vi "ExGlobalSetVar.vi"() -> ()   [LabVIEW 2010]
uses:
  Open-Close/CamHandle.vi
panel:
  in  "Value To Set":dbl format="%.2f"
  in  "Parameter ID":i32 min=0 step=1
  out "error out":errorcluster
  in  "error in (no error)":errorcluster
  # "ExGlobalSetVar:\nThis example allows the setting of a camera variable using a previously opened global camera handle."
  # "NOTICE\n\nTHIS VI USES A GLOBAL CAMERA HANDLE\n\nTHE VI EXOPENGLOBALCAM.VI MUST BE\nRUN AT THE START OF THE WORK SESSION.\nTHE CAMERA WILL REMAIN OPENED.\n\nTHE VI EXCLOSEGLOBALCAM.VI MUST\nBE RUN BEFORE LEAVING LABVIEW."
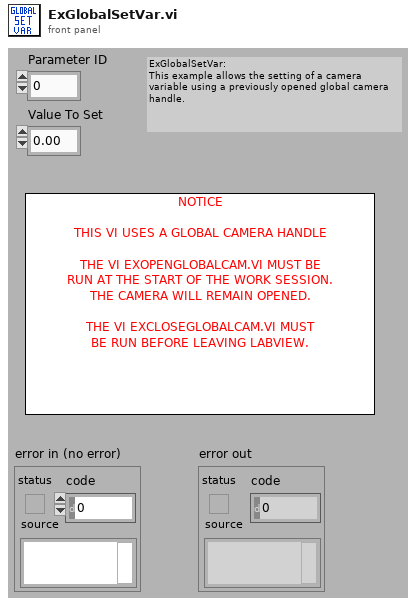
[diagram p1: front panel]
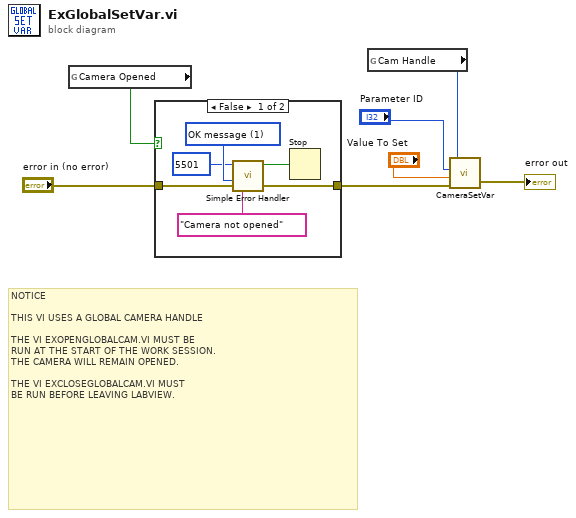
[diagram p0: block diagram]
diagram:
  # "NOTICE\n\nTHIS VI USES A GLOBAL CAMERA HANDLE\n\nTHE VI EXOPENGLOBALCAM.VI MUST BE\nRUN AT THE START OF THE WORK SESSION.\nTHE CAMERA WILL REMAIN OPENED.\n\nTHE VI EXCLOSEGLOBALCAM.VI MUST\nBE RUN BEFORE LEAVING LABVIEW."
  n1 = global read "CamHandle.vi" "Camera Opened"() -> (w4:bool)
  n2 = case shown="False" w4 {
    tunnel: "error in (no error)" -> [w12 w14]
    tunnel: [w11 w14] -> w5
    frame False {
      w13 = u16 1 items=["no dialog", "OK message", "continue or stop message"] ("type of dialog (OK msg:1)")
      n3 = call <vilib>:"Simple Error Handler.vi"("error code (no error:0)"=5501, "error source (\" \")"="Camera not opened", "type of dialog (OK msg:1)"=w13, "error in (no error)"=w12) -> ("error?"=w9:bool, "error out"=w11:errorcluster)  [unwired: 1 in, 3 out]
      n4 = Stop(stop? (T)=w9) -> ()
    }
    frame True {
    }
  }
  n5 = global read "CamHandle.vi" "Cam Handle"() -> (w3:u32)
  n6 = call <userlib>:"CameraSetVar.vi"("error in"=w5, "Value"="Value To Set", "Parameter ID"="Parameter ID", "Camera Handle"=w3) -> ("error out"=→"error out":errorcluster)  [unwired: 1 out]
